vi "Spectrometer iHR320.vi"(8 "error in (no error)":errorcluster, 11 "Spect. iHR320 In":refnum<class "Spectrometer iHR320.lvclass">) -> (0 "error out":errorcluster, 3 "Spectr. iHR320 Out":refnum<class "Spectrometer iHR320.lvclass">)   [LabVIEW 2012, in "Spectrometer iHR320.lvclass"]
doc: "Creates the iHR 320 Spectrometer object.\n\nCan also control the TRIAX 550 if the Unique ID is set to Mono1 instead of Mono2."
uses:
  Spectrometer iHR320.lvclass
  Global/GPIB Numbers.vi
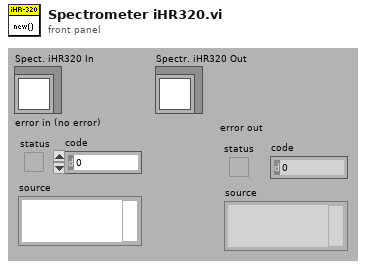
[diagram p1: front panel]
types:
  T1 = typedef "USBMono Type Def.ctl" = cluster{"Name":string, "Unique ID":string, "FW Unique ID":string}
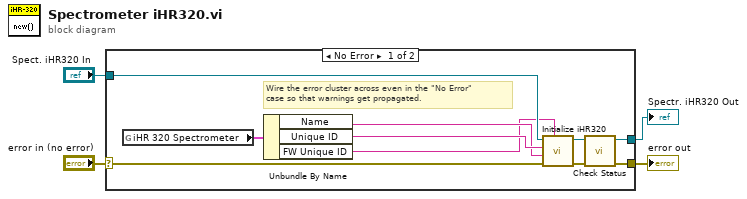
[diagram p0: block diagram]
diagram:
  n1 = case shown="No Error" "error in (no error)" {
    selector: "error in (no error)" -> [w12 w16]
    tunnel: [w8 w16] -> w2
    tunnel: [w10 w15] -> w3
    tunnel: "Spect. iHR320 In" -> [w13 w15]
    frame No Error {
      # "Wire the error cluster across even in the \"No Error\"\ncase so that warnings get propagated."
      n2 = global read "GPIB Numbers.vi" "iHR 320 Spectrometer"() -> (w14:T1)
      n3 = Unbundle By Name(w14) -> ("Name"=w6:string, "Unique ID"=w7:string, "FW Unique ID"=w5:string)
      n4 = call "Initialize iHR320.vi"("FW Unique ID"=w5, "error in (no error)"=w12, "Mono ID"=w6, "Unique ID"=w7, "Spectrometer iHR320 In"=w13) -> ("error out"=w9:errorcluster, "Spectrometer iHR320 Out"=w11:refnum<class "Spectrometer iHR320.lvclass">)  [unwired: 3 in, 2 out]
      n5 = call-dynamic "Check Status.vi"("error in (no error)"=w9, "Spectrometer iHR320 in"=w11) -> ("error out"=w8:errorcluster, "Spectrometer iHR320 out"=w10:refnum<class "Spectrometer iHR320.lvclass">)  [unwired: 6 in, 2 out]
    }
    frame Error {
    }
  }
  "error out" <- w2
  "Spectr. iHR320 Out" <- w3
